vi "Neagle_FGV.vi"(7 "Options":enum16{"Read File", "Send Array"}(ring)=enum."Send Array") -> (2 "appended array":bool[][](array[boolean]))   [LabVIEW 2015]
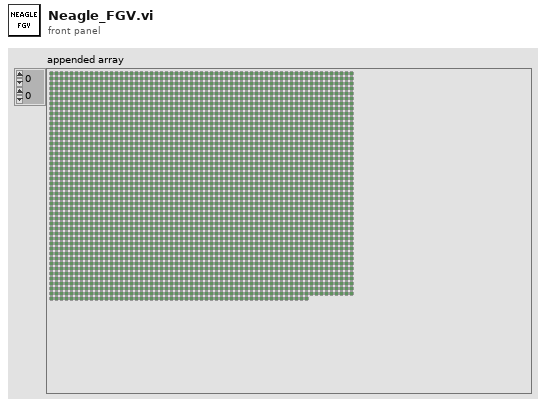
[diagram p1: front panel]
types:
  T1 = enum16{"open", "replace", "create", "open or create", "replace or create", "replace or create with confirmation"}
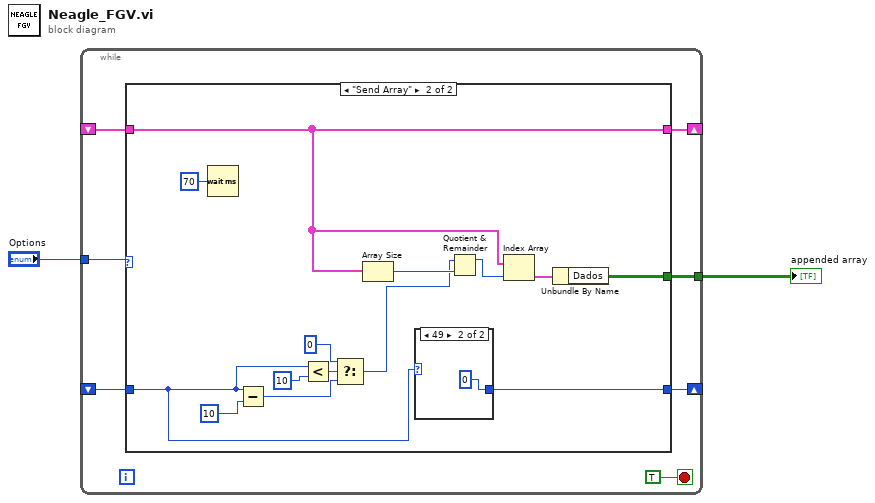
[diagram p0: block diagram]
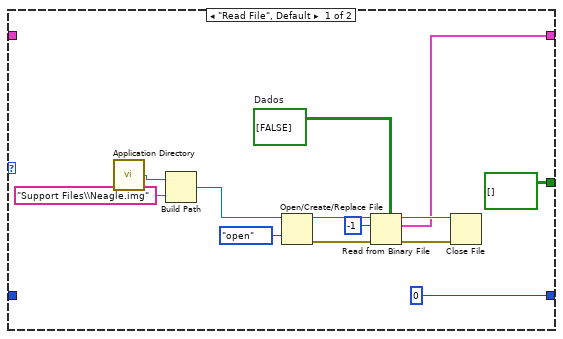
[diagram p2: hidden frame]
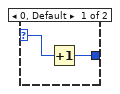
[diagram p3: hidden frame]
diagram:
  n1 = while {
    tunnel: "Options" -> [w9]
    shift-right: [w8] -> _
    shift-left: _ -> [w7]
    shift-right: [w5] -> _
    shift-left: _ -> [w4]
    tunnel: [w3] -> w1
    stop <- TRUE stop-if-true
    n2 = case shown="\"Send Array\"" w9 {
      tunnel: [w15 w33] -> w8
      tunnel: w7 -> [_ w33]
      tunnel: [0 w27] -> w5
      tunnel: w4 -> [_ w24]
      tunnel: [bool[][] [] ("Dados") w32] -> w3
      frame "Read File", Default {
        w21 = bool[][] [[FALSE]]  # Dados
        n3 = call <vilib>:"Application Directory.vi"() -> ("Application Directory"=w12:path)
        n4 = Build Path(base path=w12, name or relative path="Support Files\\Neagle.img") -> (appended path=w10:path)
        n5 = Open/Create/Replace File(file path (use dialog)=w10, operation (0:open)=T1."open") -> (refnum out=w19:refnum<file>, error out=w20:errorcluster)  [unwired: 4 in, 1 out]
        n6 = Read from Binary File(5:w21, 8:w20, 10:-1 ("count (1)"), 11:w19) -> (0:w18:errorcluster, 2:w15:cluster{"Dados":bool[][]}[], 3:w17:refnum<file>)  [unwired: 2 in, 1 out]
        n7 = Close File(refnum=w17, error in=w18) -> ()  [unwired: 2 out]
      }
      frame "Send Array" {
        n8 = Wait (ms)(milliseconds to wait=u32 70) -> ()  [unwired: 1 out]
        n9 = Subtract(x=w24, y=10) -> (x-y=w26:i32)
        n10 = Less?(x=w24, y=10) -> (x < y?=w31:bool)
        n11 = Select(t=0 ("y"), s=w31, f=w26) -> (s? t:f=w25:i32)
        n12 = Array Size(array=w33) -> (size(s)=w34:i32)
        n13 = case shown="49" w24 {
          selector: w24 -> [w38 _]
          tunnel: [w37 0 ("y")] -> w27
          frame 0, Default {
            n14 = Increment(x=w38) -> (x+1=w37:i32)
          }
          frame 49 {
          }
        }
        n15 = Quotient & Remainder(x=w25, y=w34) -> (x-y*floor(x/y)=w36:i32)  [unwired: 1 out]
        n16 = Index Array(array=w33, index=w36) -> (element=w35:cluster{"Dados":bool[][]})
        n17 = Unbundle By Name(w35) -> ("Dados"=w32:bool[][])
      }
    }
  }
  "appended array" <- w1
